vi "UHR-Fleezers Control (host) -Leonardo 04-2018 V2_sym.vi"(0 "Tab Control":T5(tab)=enum."Trap Control (RF)") -> ()   [LabVIEW 2013] (continued)
                tunnel: [w2118 w2123] -> w2110
                tunnel: w2109 -> [w2121 _]
                tunnel: w2108 -> [w2120 _]
                tunnel: w2107 -> [w2119 _]
                tunnel: w2106 -> [w2118 _]
                frame False {
                }
                frame True {
                  n1368 = Unbundle(w2131) -> (w2130:T34)
                  n1369 = call "isclickinwindow.vi"("Image Param"=w2130, "Point32"=w2129) -> ("Y px"=w2123:i32, "Height"=w2124:i32, "X px"=w2125:i32, "Width"=w2126:i32, "In image?"=w2128:bool)  [unwired: 1 in]
                  n1370 = Not(x=w2128) -> (.not. x?=w2127:bool)
                }
              }
            }
            n1371 = Not(x=w2081) -> (.not. x?=w2080:bool)
            n1372 = case shown="True" w2080 {
              tunnel: w2078 -> [_ w2144]
              tunnel: w2076 -> [_ w2143]
              tunnel: w2079 -> [_ w2142]
              tunnel: w2077 -> [_ w2141]
              frame False {
              }
              frame True {
                w2137 = FALSE ("Get Point")
                n1373 = local read "Scan lines (y)"() -> (w2146:u64)
                n1374 = local read "Actual MCL Inc (V)"() -> (w2138:dbl)
                n1375 = local read "Scan steps (MCL)"() -> (w2145:u64)
                n1376 = Divide "Y Pix/step"(x=w2141, y=w2146) -> (x/y=w2153:dbl)
                n1377 = Divide "Y V/pix"(x=w2138, y=w2153) -> (x/y=w2152:dbl)
                n1378 = Divide "Y half step offset"(x=w2138, y=2.0) -> (x/y=w2154:dbl)
                n1379 = Divide "X pix/step"(x=w2142, y=w2145) -> (x/y=w2151:dbl)
                n1380 = Negate(x=w2154) -> (-x=w2155:dbl)
                n1381 = local read "Initial Y"() -> (w2161:dbl)
                n1382 = Multiply(x=w2143, y=w2152) -> (x*y=w2162:dbl)
                n1383 = Divide "X half step offset"(x=w2138, y=2.0) -> (x/y=w2148:dbl)
                n1384 = Divide "X V/pix"(x=w2138, y=w2151) -> (x/y=w2150:dbl)
                n1385 = Multiply(x=w2138, y=w2145) -> (x*y=w2157:dbl)
                n1386 = Compound Arithmetic op=ADD(w2155, w2162, w2161) -> (w2139:dbl)
                "Pointer Y (V)" <- w2139
                n1387 = Multiply(x=w2150, y=w2144) -> (x*y=w2159:dbl)
                n1388 = Negate(x=w2148) -> (-x=w2147:dbl)
                n1389 = local read "Initial X"() -> (w2160:dbl)
                n1390 = Negate(x=w2159) -> (-x=w2158:dbl)
                n1391 = Compound Arithmetic op=ADD(w2147, w2157, w2160, w2158) -> (w2140:dbl)
                "Pointer X (V)" <- w2140
                n1392 = Or(x="Set X Only", y="Set Confocal Spot (X-Y)") -> (x .or. y?=w2133:bool)
                n1393 = Or(x="Set Confocal Spot (X-Y)", y="Set Y Only") -> (x .or. y?=w2132:bool)
                n1394 = case shown="True" w2133 {
                  tunnel: w2140 -> [_ w2163]
                  frame False {
                  }
                  frame True {
                    n1395 = property on="AO2" class="Slide (strict)"("Val(Sgnl)"=w2163) -> ()  [unwired: 2 in, 2 out]
                  }
                }
                n1396 = case shown="True" w2132 {
                  tunnel: w2139 -> [_ w2164]
                  frame False {
                  }
                  frame True {
                    n1397 = property on="AO1" class="Slide (strict)"("Val(Sgnl)"=w2164) -> ()  [unwired: 2 in, 2 out]
                  }
                }
                n1398 = local write "Set Confocal Spot (X-Y)"(w2137) -> ()
                n1399 = local write "Set X Only"(w2137) -> ()
                n1400 = local write "Set Y Only"(w2137) -> ()
              }
            }
          }
          frame 3 {
            n1401 = local read "BD 2 Frequency 1 (MHz)"() -> (w2165:dbl)
            n1402 = local read "BD 1 Frequency 1 (MHz)"() -> (w2166:dbl)
            n1403 = local write "Manipulating Trap"(TRUE ("Manipulating Trap")) -> ()
            n1404 = local write "Coords"(T8 {"Horizontal"=0, "Vertical"=0} ("Coords")) -> ()
            n1405 = while {
              tunnel: w2171 -> [w2176]
              tunnel: w2169 -> [w2175]
              tunnel: w2167 -> [w2174]
              tunnel: w2166 -> [w2173]
              tunnel: w2165 -> [w2172]
              stop <- w2177 stop-if-true
              n1406 = event shown="[0] \"Pane\": Mouse Move" {
                selector: _ -> [_ _]
                dyn-events: _ -> [_ _]
                timeout: _ -> [_ _]
                tunnel: ["Force Manip Abort" w2241] -> w2177
                tunnel: w2176 -> [w2184 _]
                tunnel: w2175 -> [w2182 _]
                tunnel: w2174 -> [w2181 _]
                tunnel: w2173 -> [w2180 _]
                tunnel: w2172 -> [w2179 _]
                event Mouse Move {
                  n1407 = event-data() -> ("Time"=w2185:u32, "Coords"=w2186:T8)  [unwired: 3 out]
                  n1408 = Less?(x=w2185, y=w2184) -> (x < y?=w2183:bool)
                  n1409 = case "Makes sure old motion events prior to mouse click aren't used" shown="False" w2183 {
                    tunnel: w2186 -> [w2228 _]
                    tunnel: w2182 -> [w2229 _]
                    tunnel: w2181 -> [w2206 _]
                    tunnel: w2180 -> [w2202 _]
                    tunnel: w2179 -> [w2201 _]
                    frame False {
                      n1410 = Subtract(x=w2228, y=w2229) -> (x-y=w2227:T8)
                      "Coords" <- w2227
                      n1411 = local read "Y RF Frequency Limits (MHz)"() -> (w2187:T16)
                      n1412 = To Double Precision Float(number=w2227) -> (double precision float=w2226:cluster{"Horizontal":dbl, "Vertical":dbl})
                      n1413 = Multiply(x=cluster{"Horizontal":dbl, "Vertical":dbl} {"Horizontal"=-1.0, "Vertical"=1.0}, y="Manipulation Scaling") -> (x*y=w2222:cluster{"Horizontal":dbl, "Vertical":dbl})
                      n1414 = local read "X RF Frequency Limits (MHz)"() -> (w2188:T16)
                      n1415 = Multiply(x=w2226, y=w2222) -> (x*y=w2224:cluster{"Horizontal":dbl, "Vertical":dbl})
                      n1416 = Unbundle By Name(w2224) -> ("Horizontal"=w2219:dbl, "Vertical"=w2223:dbl)
                      n1417 = Unbundle By Name(w2187) -> ("Maximum"=w2190:dbl, "Minimum"=w2189:dbl)
                      n1418 = Boolean To (0,1)(Boolean="Manip. X?") -> (0, 1=w2217:i16)
                      n1419 = Boolean To (0,1)(Boolean="Manip. Y?") -> (0, 1=w2214:i16)
                      n1420 = local read "BD 1 Frequency 2 (MHz)"() -> (w2204:dbl)
                      n1421 = Multiply(x=w2223, y=w2214) -> (x*y=w2216:dbl)
                      n1422 = Multiply(x=w2217, y=w2219) -> (x*y=w2220:dbl)
                      n1423 = local read "BD 2 Frequency 2 (MHz)"() -> (w2203:dbl)
                      n1424 = Unbundle By Name(w2188) -> ("Maximum"=w2192:dbl, "Minimum"=w2191:dbl)
                      n1425 = Add(x=w2201, y=w2216) -> (x+y=w2194:dbl)
                      n1426 = Add(x=w2202, y=w2220) -> (x+y=w2196:dbl)
                      n1427 = In Range and Coerce(upper limit=w2192, x=w2196, lower limit=w2191) -> (coerced(x)=w2195:dbl)  [unwired: 1 out]
                      n1428 = In Range and Coerce(upper limit=w2190, x=w2194, lower limit=w2189) -> (coerced(x)=w2193:dbl)  [unwired: 1 out]
                      n1429 = Subtract(x=w2195, y=w2204) -> (x-y=w2213:dbl)
                      n1430 = Subtract(x=w2193, y=w2203) -> (x-y=w2212:dbl)
                      n1431 = Square(x=w2213) -> (x^2=w2211:dbl)
                      n1432 = Square(x=w2212) -> (x^2=w2210:dbl)
                      n1433 = Add(x=w2211, y=w2210) -> (x+y=w2209:dbl)
                      n1434 = Square Root(x=w2209) -> (sqrt(x)=w2205:dbl)
                      n1435 = In Range and Coerce(upper limit="Limit Max (MHz)", x=w2205, lower limit="Limit Min (MHz)") -> (In Range?=w2198:bool)  [unwired: 1 out]
                      n1436 = Not(x="Limits Enable") -> (.not. x?=w2197:bool)
                      n1437 = Or(x=w2198, y=w2197) -> (x .or. y?=w2199:bool)
                      n1438 = case shown="True" w2199 {
                        tunnel: w2206 -> [_ w2239]
                        tunnel: w2205 -> [_ w2230]
                        tunnel: w2195 -> [_ w2237]
                        tunnel: w2204 -> [_ w2236]
                        tunnel: w2193 -> [_ w2235]
                        tunnel: w2203 -> [_ w2234]
                        tunnel: w2188 -> [_ w2232]
                        tunnel: w2187 -> [_ w2231]
                        frame False {
                        }
                        frame True {
                          n1439 = local read "BD 1 Frequency 3 (MHz)"() -> (w2238:dbl)
                          n1440 = local read "BD 2 Frequency 3 (MHz)"() -> (w2233:dbl)
                          n1441 = local write "Trap Delta (MHz)"(w2230) -> ()
                          n1442 = property on="Initial delta (MHz)" class="DigNum (strict)"("Val(Sgnl)"=w2230) -> ()  [unwired: 2 in, 2 out]
                          n1443 = call "set RF board frequency - interlace.vi"("Board 2 Frequency Limits"=w2231, "Board 1 Frequency Limits"=w2232, "FPGA VI Reference In"=w2239, "Board 2 Frequency 3 (MHz)"=w2233, "Board 1 Frequency 3 (MHz)"=w2238, "Board 2 Frequency 2 (MHz)"=w2234, "Board 2 Frequency 1 (MHz)"=w2235, "Board 1 Frequency 2 (MHz)"=w2236, "Board 1 Frequency 1  (MHz)"=w2237) -> ()  [unwired: 1 in, 2 out]
                          n1444 = local write "BD 2 Frequency 1 (MHz)"(w2235) -> ()
                          n1445 = local write "BD 1 Frequency 1 (MHz)"(w2237) -> ()
                        }
                      }
                    }
                    frame True {
                    }
                  }
                }
                event Mouse Up {
                  n1446 = event-data() -> ("Button"=w2240:u16)  [unwired: 8 out]
                  n1447 = case shown="3" w2240 {
                    tunnel: [FALSE TRUE] -> w2241
                    frame 0, Default {
                    }
                    frame 3 {
                      n1448 = local write "Manipulating Trap"(FALSE ("Manipulating Trap")) -> ()
                    }
                  }
                }
              }
            }
          }
        }
      }
      event Mouse Move {
        n1449 = event-data() -> ()  [unwired: 6 out]
      }
    }
    n1450 = local read "Stop All"() -> (w2062:bool)
    n1451 = node-c288() -> ()  [unwired: 2 out]
  }
  n1452 = node-c288(w53) -> ()  [unwired: 1 out]
  n1453 = node-c288(w102) -> ()  [unwired: 1 out]
  n1454 = node-c288(w109) -> ()  [unwired: 1 out]
  n1455 = node-c288(i64 1 ("Period"), 1 ("Processor")) -> (w195:T25)  [unwired: 2 out]
  n1456 = timed-loop "Acquire Data" {
    tunnel: w61 -> [w2550]
    tunnel: w76 -> [w2549]
    tunnel: [w2580] -> w69
    tunnel: [w2574] -> w2
    timing: w195 -> [_]
    timing-out: [_] -> w194
    tunnel: w93 -> [w2396]
    stop <- "Stop All" stop-if-true
    (unwired) u32 0 ("Number of Elements")
    w2383 = "NI_ChannelName" ("name")
    n1457 = node-c288() -> ()  [unwired: 2 out]
    n1458 = First Call?() -> (First Call?: T/F=w2349:bool)
    n1459 = Or(x="Reset", y=w2349) -> (x .or. y?=w2350:bool)
    n1460 = local read "MCL Tracking"() -> (w2287:bool)
    n1461 = case "Reset data stream" shown="True" w2350 {
      tunnel: w2550 -> [w2700 w2708]
      tunnel: w2549 -> [w2699 w2707]
      tunnel: [w2700 w2702] -> w2285
      tunnel: [w2699 w2701] -> w2545
      frame False {
      }
      frame True {
        w2705 = TRUE ("AI to FIFO")
        n1462 = local write "Overflow (data lost)"(FALSE ("Overflow (data lost)")) -> ()
        n1463 = call "reset FPGA DMA.vi"("error in"=w2707, "FPGA VI Reference In"=w2708) -> ("error out"=w2703:errorcluster, "FPGA VI Reference Out"=w2704:T20)
        n1464 = xnode "Read/Write Control"("FPGA VI Reference In"=w2704, "error in"=w2703, "AI to FIFO"=w2705, "APD to FIFO"=w2705) -> ("FPGA VI Reference Out"=w2702:T20, "error out"=w2701:errorcluster)
      }
    }
    n1465 = Or(x="Start AOD Scan", y="Trap Raster Scan") -> (x .or. y?=w2503:bool)
    n1466 = case "Start AOM raster scan" shown="True" w2503 {
      tunnel: w2285 -> [w3441 w3452]
      tunnel: w2545 -> [w3440 w3451]
      tunnel: [w3441 w3445] -> w2284
      tunnel: [w3440 w3444] -> w2544
      frame False {
      }
      frame True {
        n1467 = case shown="True" "Restart DMA? (AOD)" {
          tunnel: [w3492 w3494] -> w3446
          tunnel: [w3491 w3493] -> w3447
          tunnel: w3452 -> [w3492 w3496]
          tunnel: w3451 -> [w3491 w3495]
          frame False {
          }
          frame True {
            n1468 = local write "Overflow (data lost)"(FALSE ("Overflow (data lost)")) -> ()
            n1469 = call "reset FPGA DMA.vi"("error in"=w3495, "FPGA VI Reference In"=w3496) -> ("error out"=w3493:errorcluster, "FPGA VI Reference Out"=w3494:T20)
          }
        }
        n1470 = local write "Trap Raster Scan"(FALSE ("Trap Raster Scan")) -> ()
        n1471 = case shown="False" "Move MCL Also?" {
          tunnel: w3447 -> [w3456 w3486]
          tunnel: w3446 -> [w3457 w3487]
          tunnel: [w3455 w3490] -> w3445
          tunnel: [w3454 w3489] -> w3444
          tunnel: "Raster to target force?" -> [w3453 w3459]
          frame False {
            w3458 = TRUE ("AI to FIFO")
            n1472 = xnode "Read/Write Control"("FPGA VI Reference In"=w3457, "error in"=w3456, "AI to FIFO"=w3458, "APD to FIFO"=w3458, "Start scan"=w3458, "Raster to target force"=w3453) -> ("FPGA VI Reference Out"=w3455:T20, "error out"=w3454:errorcluster)
          }
          frame True {
            w3483 = FALSE ("1D or 2D Scan?")
            w3488 = TRUE ("AI to FIFO")
            # "Count for MCL loop"
            # "N total cycles"
            # "N steps"
            # "V_int"
            n1473 = local read "Scan Range (nm)"() -> (w3465:dbl)
            n1474 = local read "Number of F/B Scans (AOD)"() -> (w3482:u16)
            n1475 = Sign(1:w3465) -> (0:w3464:dbl)
            n1476 = Compound Arithmetic op=MULTIPLY(w3465, "MCL Step Position Ratio", "MCL/AOM Scale Tweak") -> (w3469:dbl)
            n1477 = Negate(x=w3464) -> (-x=w3461:dbl)
            n1478 = Multiply(x=w3461, y="MCL Step Increment (V_int)") -> (x*y=w3463:dbl)
            n1479 = Divide(x=w3469, y="MCL X Cal (nm/V)") -> (x/y=w3475:dbl)
            n1480 = Multiply(x=32767.0 ("y"), y=w3475) -> (x*y=w3481:dbl)
            n1481 = local read "Total Counts (ticks)"() -> (w3466:u32)
            n1482 = local read "Cycles/step (AOD)"() -> (w3477:u64)
            n1483 = local read "Scan steps (AOD)"() -> (w3478:u64)
            n1484 = Divide(x=w3481, y=10.0) -> (x/y=w3474:dbl)
            n1485 = Divide(x=w3474, y="MCL Step Increment (V_int)") -> (x/y=w3472:dbl)
            n1486 = Absolute Value(x=w3472) -> (abs(x)=w3460:dbl)
            n1487 = Compound Arithmetic op=MULTIPLY(w3478, w3477, w3466) -> (w3473:u64)
            n1488 = local write "wait to reset values"(w3488) -> ()
            n1489 = local write "MCL Scanning"(w3488) -> ()
            n1490 = Divide(x=w3473, y=w3460) -> (x/y=w3470:dbl)
            "MCL Count" <- w3470
            n1491 = xnode "Read/Write Control"("FPGA VI Reference In"=w3487, "error in"=w3486, "Scan steps (MCL)"=w3460, "Number of scans (MCL)"=w3482, "Cycles per step (MCL)"=u64 1, "Scan freq.  increment (MCL)"=w3463, "1D or 2D Scan?"=w3483, "MCL Scan Axis"=w3483, "Cont. Scan (MCL)"=w3483, "MCL count"=w3470) -> ("FPGA VI Reference Out"=w3485:T20, "error out"=w3484:errorcluster)
            n1492 = xnode "Read/Write Control"("FPGA VI Reference In"=w3485, "error in"=w3484, "AI to FIFO"=w3488, "APD to FIFO"=w3488, "Start scan"=w3488, "Start scan (MCL)"=w3488, "Raster to target force"=w3459) -> ("FPGA VI Reference Out"=w3490:T20, "error out"=w3489:errorcluster)
          }
        }
        "Raster Scanning..." <- TRUE ("Scanning...")
      }
    }
    n1493 = And(x="Save scans", y=w2503) -> (x .and. y?=w2543:bool)
    n1494 = Compound Arithmetic op=OR("Start MCL Scan", "Confocal Image", "Confocal Linescan") -> (w2501:bool)
    n1495 = And(x="Save Data (MCL)", y=w2501) -> (x .and. y?=w2542:bool)
    n1496 = case "Start MCL raster scan" shown="True" w2501 {
      tunnel: w2284 -> [w2991 w3006]
      tunnel: w2544 -> [w2990 w3005]
      tunnel: [w2991 w3001] -> w2319
      tunnel: [w2990 w3000] -> w2318
      tunnel: [FALSE w2999] -> w2528
      tunnel: "Start MCL Scan" -> [_ w2994]
      tunnel: "Confocal Image" -> [_ w2993]
      tunnel: "Confocal Linescan" -> [_ _]
      frame False {
      }
      frame True {
        w2999 = TRUE
        n1497 = case shown="True" "Restart DMA? (MCL)" {
          tunnel: [w3051 w3053] -> w3004
          tunnel: [w3050 w3052] -> w3003
          tunnel: w3006 -> [w3051 w3056]
          tunnel: w3005 -> [w3050 w3055]
          frame False {
          }
          frame True {
            n1498 = call "reset FPGA DMA.vi"("error in"=w3055, "FPGA VI Reference In"=w3056) -> ("error out"=w3052:errorcluster, "FPGA VI Reference Out"=w3053:T20)
            n1499 = local write "Overflow (data lost)"(FALSE ("Overflow (data lost)")) -> ()
          }
        }
        n1500 = case shown="False" w2994 {
          selector: w2994 -> [_ w3010]
          tunnel: w2993 -> [w3009 _]
          tunnel: [w3009 w3010] -> w2992
          frame False {
            n1501 = property on="2D or 1D Scan" class="Bool (strict)"("Val(Sgnl)"=w3009) -> ()  [unwired: 2 in, 2 out]
            n1502 = property on="Confocal Image" class="Bool (strict)"("Value"=FALSE ("Start Confocal Map")) -> ()  [unwired: 2 in, 2 out]
          }
          frame True {
          }
        }
        n1503 = local write "MCL Scanning"(w2999) -> ()
        n1504 = local read "AO1"() -> (w2996:dbl)
        n1505 = local read "AO2"() -> (w2995:dbl)
        n1506 = case shown="True" "Center Scan" {
          tunnel: w3004 -> [w3017 w3049]
          tunnel: w3003 -> [w3016 w3048]
          tunnel: [w3015 w3047] -> w3001
          tunnel: [w3014 w3046] -> w3000
          tunnel: [w3012 w3033] -> w2998
          tunnel: [w3011 w3032] -> w2997
          tunnel: w2996 -> [w3012 w3038]
          tunnel: w2995 -> [w3011 w3041]
          tunnel: w2992 -> [_ _]
          frame False {
            w3013 = TRUE ("AI to FIFO")
            n1507 = xnode "Read/Write Control"("FPGA VI Reference In"=w3017, "error in"=w3016, "AI to FIFO"=w3013, "APD to FIFO"=w3013, "Start scan (MCL)"=w3013) -> ("FPGA VI Reference Out"=w3015:T20, "error out"=w3014:errorcluster)
          }
          frame True {
            w3045 = TRUE ("AI to FIFO")
            n1508 = local read "Scan steps (MCL)"() -> (w3024:u64)
            n1509 = local read "Scan lines (y)"() -> (w3020:u64)
            n1510 = local read "Fast Scan Dir"() -> (w3031:bool)
            n1511 = local read "Actual MCL Inc (V)"() -> (w3021:dbl)
            n1512 = Decrement(x=w3020) -> (x-1=w3019:u64)
            n1513 = Decrement(x=w3024) -> (x-1=w3023:u64)
            n1514 = Multiply(x=w3021, y=w3019) -> (x*y=w3018:dbl)
            n1515 = Divide(x=w3018, y=2.0) -> (x/y=w3028:dbl)
            n1516 = Multiply(x=w3021, y=w3023) -> (x*y=w3022:dbl)
            n1517 = Divide(x=w3022, y=2.0) -> (x/y=w3027:dbl)
            n1518 = Select(t=w3027, s=w3031, f=w3028) -> (s? t:f=w3026:dbl)
            n1519 = Select(t=w3028, s=w3031, f=w3027) -> (s? t:f=w3030:dbl)
            n1520 = Subtract(x=w3038, y=w3030) -> (x-y=w3029:dbl)
            n1521 = Subtract(x=w3041, y=w3026) -> (x-y=w3025:dbl)
            n1522 = local read "2D or 1D Scan"() -> (w3043:bool)
            n1523 = Not(x=w3031) -> (.not. x?=w3037:bool)
            n1524 = Not(x=w3043) -> (.not. x?=w3039:bool)
            n1525 = And(x=w3031, y=w3039) -> (x .and. y?=w3040:bool)
            n1526 = And(x=w3039, y=w3037) -> (x .and. y?=w3042:bool)
            n1527 = Select(t=w3041, s=w3042, f=w3025) -> (s? t:f=w3032:dbl)
            n1528 = Select(t=w3038, s=w3040, f=w3029) -> (s? t:f=w3033:dbl)
            n1529 = call "Volt to I16.vi"("Voltage In"=w3033) -> ("I16 Voltage Out"=w3036:i16)
            n1530 = call "Volt to I16.vi"("Voltage In"=w3032) -> ("I16 Voltage Out"=w3035:i16)
            n1531 = xnode "Read/Write Control"("FPGA VI Reference In"=w3049, "error in"=w3048, "AI to FIFO"=w3045, "APD to FIFO"=w3045, "Start scan (MCL)"=w3045, "AO1 (Y)"=w3036, "AO2 (X)"=w3035) -> ("FPGA VI Reference Out"=w3047:T20, "error out"=w3046:errorcluster)
          }
        }
        "Initial Y" <- w2998
        "Initial X" <- w2997
        "wait to reset values" <- w2999
      }
    }
    n1532 = local read "Trap Pos Elements/DMA read"() -> (w2392:u32)
    n1533 = local read "Trap AI Elements/DMA read"() -> (w2317:u32)
    n1534 = local read "APD Elements/DMA read"() -> (w2431:u32)
    n1535 = local read "Trap AI FIFO Depth"() -> (w2590:u32)
    n1536 = xnode "Invoke Method"("FPGA VI Reference In"=w2319, "error in"=w2318, "Number of Elements"=w2392, "Timeout (ms)"=-1) -> ("Data"=w2356:u16[], "Elements Remaining"=→"Trap Pos FIFO El Remaining":u32)  [unwired: 2 out]
    n1537 = xnode "Invoke Method"("FPGA VI Reference In"=w2319, "error in"=w2318, "Number of Elements"=w2317, "Timeout (ms)"=-1 ("Timeout")) -> ("FPGA VI Reference Out"=w2288:T20, "error out"=w2320:errorcluster, "Data"=w2316:i16[], "Elements Remaining"=w2321:u32)
    "Trap AI FIFO El. Rem." <- w2321
    n1538 = xnode "Get APD Data"("FPGA VI Reference In"=w2319, "error in"=w2318, "Number of Elements"=w2431, "Timeout (ms)"=-1) -> ("Data"=w2430:u32[], "Elements Remaining"=→"APD FIFO Elements Remaining":u32)  [unwired: 2 out]
    n1539 = Subtract(x=w2590, y=w2317) -> (x-y=w2589:u32)
    n1540 = Decimate 1D Array(w2356) -> (w2353:u16[], w2355:u16[], w2354:u16[])
    n1541 = Divide(x=w2321, y=w2589) -> (x/y=w2588:dbl)
    "Buffer Status" <- w2588
    n1542 = To Unsigned Long Integer(number=w2353) -> (unsigned 32bit integer=w2352:u32[])
    n1543 = Join Numbers(hi=w2355, lo=w2354) -> ((hi.lo)=w2351:u32[])
    n1544 = Equal?(x=w2588, y=1.0) -> (x = y?=w2586:bool)
    n1545 = Join Numbers(hi=w2352, lo=w2351) -> ((hi.lo)=w2345:u64[])
    n1546 = call "IR AOM word to freq - vec.vi"("Frequency Word In (double vec)"=w2345) -> ("Frequency Out"=w2391:dbl[])
    n1547 = case "Alert buffer overflow" shown="True" w2586 {
      frame False {
      }
      frame True {
        n1548 = call <vilib>:"Beep.vi"() -> ()  [unwired: 3 in, 9 out]
        "Overflow (data lost)" <- TRUE ("Overflow (data lost)")
      }
    }
    n1549 = Decimate 1D Array(w2391) -> (w2390:dbl[], w2389:dbl[])
    n1550 = Array Size(array=w2316) -> (size(s)=→"Waveform Chart":i32)
    n1551 = Build Array(w2390, w2389) -> (w2388:dbl[][])
    n1552 = local read "Trap Sets"() -> (w2463:u32)
    n1553 = case "Deinterlace trap data, average down PSD" shown="2" w2463 {
      tunnel: w2316 -> [w3086 w3151]
      tunnel: [w3083 w3148] -> w2456
      tunnel: [w3086 w3150] -> w2348
      tunnel: "Detector Type" -> [w3085 w3146]
      tunnel: [w3084 w3149] -> w2455
      tunnel: [w3082 w3147] -> w2561
      frame 1, Default {
        n1554 = Divide(x=w3086, y=3276.7) -> (x/y=w3087:dbl[])
        n1555 = Decimate 1D Array(w3087) -> (w3096:dbl[], w3095:dbl[], w3094:dbl[], w3093:dbl[], w3092:dbl[], w3091:dbl[], w3090:dbl[], w3089:dbl[])
        n1556 = case shown="\"IR-QPD + PSD + FB-QPD position\"" w3085 {
          tunnel: w3096 -> [w3120 w3145]
          tunnel: w3095 -> [w3119 w3144]
          tunnel: w3094 -> [w3104 w3122]
          tunnel: w3093 -> [w3105 w3132]
          tunnel: w3092 -> [w3118 w3143]
          tunnel: w3091 -> [w3117 w3142]
          tunnel: w3090 -> [w3101 w3123]
          tunnel: w3089 -> [w3100 w3121]
          tunnel: [w3099 w3129] -> w3084
          tunnel: [w3098 w3128] -> w3083
          tunnel: [w3097 w3127] -> w3082
          frame "IR-QPD + PSD + FB-QPD", Default {
            w3097 = 0  # Channel pattern
            n1557 = Divide(x=w3120, y=w3105) -> (x/y=w3107:dbl[])
            n1558 = Divide(x=w3119, y=w3105) -> (x/y=w3106:dbl[])
            n1559 = Divide(x=w3118, y=w3101) -> (x/y=w3103:dbl[])
            n1560 = Divide(x=w3117, y=w3100) -> (x/y=w3102:dbl[])
            n1561 = Build Array(w3107, w3106, w3105, w3104, w3103, w3102, w3101, w3100) -> (w3098:dbl[][])
            n1562 = Bundle("T1 Y", "T1 X", "T1 Sum", "FB Sum", "PSD Y", "PSD X", "PSD Y Sum", "PSD X Sum") -> (w3116:T42)  [unwired: 1 out]
            n1563 = Cluster To Array(cluster=w3116) -> (array=w3099:string[])
          }
          frame "IR-QPD + PSD + FB-QPD position" {
            w3127 = 3  # Channel pattern
            n1564 = Negate(x=w3123) -> (-x=w3124:dbl[])
            n1565 = Divide(x=w3145, y=w3132) -> (x/y=w3134:dbl[])
            n1566 = Divide(x=w3144, y=w3132) -> (x/y=w3133:dbl[])
            n1567 = Divide(x=w3143, y=w3123) -> (x/y=w3131:dbl[])
            n1568 = Divide(x=w3142, y=w3124) -> (x/y=w3130:dbl[])
            n1569 = Build Array(w3134, w3133, w3132, w3121, w3122, w3131, w3130, w3123) -> (w3128:dbl[][])
            n1570 = Bundle("T1 Y", "T1 X", "T1 Sum", "FB X", "FB Sum", "PSD Y", "PSD X", "PSD Y Sum") -> (w3141:T42)  [unwired: 1 out]
            n1571 = Cluster To Array(cluster=w3141) -> (array=w3129:string[])
          }
        }
      }
      frame 2 {
        n1572 = case shown="\"UCB Fleezers 052511\"" w3146 {
          tunnel: w3151 -> [w3213 w3280 w3319 w3419]
          tunnel: [w3152 w3272 w3315 w3350] -> w3150
          tunnel: [w3179 w3263 w3317 w3397] -> w3149
          tunnel: [w3178 w3227 w3308 w3364] -> w3148
          tunnel: [w3172 w3262 w3349 w3395] -> w3147
          frame "IR-QPD + PSD + FB-QPD", Default {
            w3172 = 1  # Channel pattern
            # "time average x2 the 4th signal and the 4 psd signals (detection laser)"
            # "deinterlace 3 signals from qpd"
            n1573 = Decimate 1D Array(w3213) -> (w3212:i16[], w3211:i16[], w3177:i16[], w3210:i16[], w3200:i16[], w3198:i16[], w3197:i16[], w3195:i16[])
            n1574 = call "downsample 1D array - double.vi"("Ave N"=2.0, "Array In"=w3200) -> ("Array Out"=w3199:dbl[])  [unwired: 1 out]
            n1575 = call "downsample 1D array - double.vi"("Ave N"=2.0, "Array In"=w3195) -> ("Array Out"=w3194:dbl[])  [unwired: 1 out]
            n1576 = call "downsample 1D array - double.vi"("Ave N"=2.0, "Array In"=w3197) -> ("Array Out"=w3196:dbl[])  [unwired: 1 out]
            n1577 = call "downsample 1D array - double.vi"("Ave N"=2.0, "Array In"=w3198) -> ("Array Out"=w3180:dbl[])  [unwired: 1 out]
            n1578 = Decimate 1D Array(w3212) -> (w3209:i16[], w3181:i16[])
            n1579 = Decimate 1D Array(w3211) -> (w3208:i16[], w3206:i16[])
            n1580 = Decimate 1D Array(w3210) -> (w3207:i16[], w3205:i16[])
            n1581 = Decimate 1D Array(w3177) -> (w3176:i16[], w3175:i16[])
            n1582 = Interleave 1D Arrays(w3209, w3208, w3207, w3181, w3206, w3205, w3176, w3175, w3199, w3180, w3196, w3194) -> (w3193:dbl[])
            n1583 = To Word Integer(number=w3193) -> (16bit integer=w3152:i16[])
            n1584 = Divide(x=w3193, y=3276.7) -> (x/y=w3192:dbl[])
            n1585 = Decimate 1D Array(w3192) -> (w3191:dbl[], w3190:dbl[], w3189:dbl[], w3188:dbl[], w3187:dbl[], w3186:dbl[], w3174:dbl[], w3173:dbl[], w3185:dbl[], w3184:dbl[], w3183:dbl[], w3182:dbl[])
            n1586 = Divide(x=w3191, y=w3189) -> (x/y=w3159:dbl[])
            n1587 = Divide(x=w3190, y=w3189) -> (x/y=w3158:dbl[])
            n1588 = Divide(x=w3188, y=w3186) -> (x/y=w3157:dbl[])
            n1589 = Divide(x=w3187, y=w3186) -> (x/y=w3156:dbl[])
            n1590 = Divide(x=w3185, y=w3183) -> (x/y=w3155:dbl[])
            n1591 = Divide(x=w3184, y=w3182) -> (x/y=w3154:dbl[])
            n1592 = Bundle("T1 Y", "T1 X", "T1 Sum", "T2 Y", "T2 X", "T2 Sum", "T1 FB Sum", "T2 FB Sum", "PSD Y", "PSD X", "PSD Y Sum", "PSD X Sum") -> (w3160:T43)  [unwired: 1 out]
            n1593 = Build Array(w3159, w3158, w3189, w3157, w3156, w3186, w3174, w3173, w3155, w3154, w3183, w3182) -> (w3178:dbl[][])
            n1594 = Cluster To Array(cluster=w3160) -> (array=w3179:string[])
          }
          frame "IR-QPD + PSD + FB-QPD X position" {
            w3262 = 2  # Channel pattern
            # "convert\nADC numbers\nto volts"
            # "time average x2 the 3 psd signals (detection laser)"
            # "deinterlace 3 signals from qpds"
            n1595 = Decimate 1D Array(w3280) -> (w3279:i16[], w3278:i16[], w3215:i16[], w3216:i16[], w3225:i16[], w3222:i16[], w3219:i16[], w3250:i16[])
            n1596 = Decimate 1D Array(w3279) -> (w3277:i16[], w3264:i16[])
            n1597 = call "downsample 1D array - I16.vi"("Ave N"=2.0, "Array In"=w3225) -> ("Array Out"=w3223:i16[])  [unwired: 1 in]
            n1598 = call "downsample 1D array - I16.vi"("Ave N"=2.0, "Array In"=w3222) -> ("Array Out"=w3220:i16[])  [unwired: 1 in]
            n1599 = Decimate 1D Array(w3278) -> (w3276:i16[], w3274:i16[])
            n1600 = Decimate 1D Array(w3216) -> (w3275:i16[], w3273:i16[])
            n1601 = Decimate 1D Array(w3250) -> (w3249:i16[], w3247:i16[])
            n1602 = Decimate 1D Array(w3215) -> (w3248:i16[], w3246:i16[])
            n1603 = call "downsample 1D array - I16.vi"("Ave N"=2.0, "Array In"=w3219) -> ("Array Out"=w3217:i16[])  [unwired: 1 in]
            n1604 = Interleave 1D Arrays(w3277, w3276, w3275, w3264, w3274, w3273, w3249, w3248, w3247, w3246, w3223, w3220, w3217) -> (w3272:i16[])
            n1605 = Divide(x=w3272, y=3276.7) -> (x/y=w3271:dbl[])
            n1606 = Decimate 1D Array(w3271) -> (w3270:dbl[], w3269:dbl[], w3268:dbl[], w3267:dbl[], w3266:dbl[], w3265:dbl[], w3238:dbl[], w3236:dbl[], w3235:dbl[], w3233:dbl[], w3232:dbl[], w3231:dbl[], w3228:dbl[])
            n1607 = Divide(x=w3270, y=w3268) -> (x/y=w3254:dbl[])
            n1608 = Divide(x=w3269, y=w3268) -> (x/y=w3253:dbl[])
            n1609 = Divide(x=w3267, y=w3265) -> (x/y=w3252:dbl[])
            n1610 = Divide(x=w3266, y=w3265) -> (x/y=w3251:dbl[])
            n1611 = Divide(x=w3238, y=w3236) -> (x/y=w3237:dbl[])
            n1612 = Divide(x=w3235, y=w3233) -> (x/y=w3234:dbl[])
            n1613 = Divide(x=w3232, y=w3228) -> (x/y=w3230:dbl[])
            n1614 = Negate(x=w3228) -> (-x=w3226:dbl[])
            n1615 = Divide(x=w3231, y=w3226) -> (x/y=w3229:dbl[])
            n1616 = Bundle("T1 Y", "T1 X", "T1 Sum", "T2 Y", "T2 X", "T2 Sum", "T1 FB X", "T1 FB Sum", "T2 FB X", "T2 FB Sum", "PSD Y", "PSD X", "PSD Y Sum") -> (w3255:T44)  [unwired: 1 out]
            n1617 = Build Array(w3254, w3253, w3268, w3252, w3251, w3265, w3237, w3236, w3234, w3233, w3230, w3229, w3228) -> (w3227:dbl[][])
            n1618 = Cluster To Array(cluster=w3255) -> (array=w3263:string[])
          }
          frame "UCB Fleezers 052511" {
            w3349 = 2  # Channel pattern
            n1619 = Select(t=i16 -1, s="Negate X signals", f=i16 1) -> (s? t:f=w3289:i16)
            n1620 = Decimate 1D Array(w3319) -> (w3290:i16[], w3291:i16[], w3302:i16[], w3318:i16[], w3287:i16[], w3285:i16[], w3283:i16[], w3299:i16[])
            n1621 = Multiply(x=w3289, y=w3291) -> (x*y=w3288:i16[])
            n1622 = Decimate 1D Array(w3290) -> (w3347:i16[], w3337:i16[])
            n1623 = Decimate 1D Array(w3288) -> (w3346:i16[], w3345:i16[])
            n1624 = Decimate 1D Array(w3302) -> (w3296:i16[], w3295:i16[])
            n1625 = Decimate 1D Array(w3318) -> (w3301:i16[], w3300:i16[])
            n1626 = Decimate 1D Array(w3285) -> (w3284:i16[])  [unwired: 1 out]
            n1627 = Decimate 1D Array(w3299) -> (w3298:i16[], w3297:i16[])
            n1628 = Decimate 1D Array(w3283) -> (w3282:i16[])  [unwired: 1 out]
            n1629 = Decimate 1D Array(w3287) -> (w3286:i16[])  [unwired: 1 out]
            n1630 = Interleave 1D Arrays(w3347, w3346, w3301, w3337, w3345, w3300, w3298, w3296, w3297, w3295, w3286, w3284, w3282) -> (w3315:i16[])
            n1631 = Divide(x=w3315, y=3276.7) -> (x/y=w3344:dbl[])
            n1632 = Decimate 1D Array(w3344) -> (w3343:dbl[], w3342:dbl[], w3341:dbl[], w3340:dbl[], w3339:dbl[], w3338:dbl[], w3314:dbl[], w3312:dbl[], w3311:dbl[], w3309:dbl[], w3307:dbl[], w3304:dbl[], w3305:dbl[])
            n1633 = Divide(x=w3343, y=w3341) -> (x/y=w3324:dbl[])
            n1634 = Divide(x=w3342, y=w3341) -> (x/y=w3323:dbl[])
            n1635 = Divide(x=w3340, y=w3338) -> (x/y=w3322:dbl[])
            n1636 = Divide(x=w3339, y=w3338) -> (x/y=w3321:dbl[])
            n1637 = Divide(x=w3314, y=w3312) -> (x/y=w3313:dbl[])
            n1638 = Divide(x=w3311, y=w3309) -> (x/y=w3310:dbl[])
            n1639 = Divide(x=w3307, y=w3305) -> (x/y=w3306:dbl[])
            n1640 = Divide(x=w3304, y=w3305) -> (x/y=w3303:dbl[])
            n1641 = Build Array(w3324, w3323, w3341, w3322, w3321, w3338, w3313, w3312, w3310, w3309, w3306, w3303, w3305) -> (w3308:dbl[][])
            n1642 = Bundle("T1 Y", "T1 X", "T1 Sum", "T2 Y", "T2 X", "T2 Sum", "T1 FB X", "T2 FB Sum", "T2 FB X", "T2 FB Sum", "PSD Y", "PSD X", "PSD Sum") -> (w3325:T44)  [unwired: 1 out]
            n1643 = Cluster To Array(cluster=w3325) -> (array=w3317:string[])
          }
          frame "IR-QPD + PSD + FB-QPD XY positions" {
            w3395 = 4  # Channel pattern
            # "time average x2 the 3 psd signals (detection laser)"
            # "deinterlace 3 signals from qpds"
            n1644 = Decimate 1D Array(w3419) -> (w3418:i16[], w3417:i16[], w3396:i16[], w3416:i16[], w3362:i16[], w3408:i16[], w3407:i16[], w3384:i16[])
            n1645 = Decimate 1D Array "QPD Y"(w3418) -> (w3415:i16[], w3398:i16[])
            n1646 = call "downsample 1D array - double.vi"("Ave N"=2.0, "Array In"=w3408) -> ("Array Out"=w3383:dbl[])  [unwired: 1 out]
            n1647 = call "downsample 1D array - double.vi"("Ave N"=2.0, "Array In"=w3407) -> ("Array Out"=w3382:dbl[])  [unwired: 1 out]
            n1648 = Decimate 1D Array "Feedback Sum"(w3396) -> (w3380:i16[], w3378:i16[])
            n1649 = Decimate 1D Array "Feedback Y"(w3362) -> (w3361:i16[], w3360:i16[])
            n1650 = Decimate 1D Array "Feedback X"(w3384) -> (w3381:i16[], w3379:i16[])
            n1651 = Decimate 1D Array "QPD Sum"(w3416) -> (w3413:i16[], w3411:i16[])
            n1652 = Decimate 1D Array "QPD X"(w3417) -> (w3414:i16[], w3412:i16[])
            n1653 = Interleave 1D Arrays(w3415, w3414, w3413, w3398, w3412, w3411, w3361, w3381, w3380, w3360, w3379, w3378, w3383, w3382) -> (w3406:dbl[])
            n1654 = To Word Integer(number=w3406) -> (16bit integer=w3350:i16[])
            n1655 = Divide(x=w3406, y=3276.7) -> (x/y=w3405:dbl[])
            n1656 = Decimate 1D Array(w3405) -> (w3404:dbl[], w3403:dbl[], w3402:dbl[], w3401:dbl[], w3400:dbl[], w3399:dbl[], w3357:dbl[], w3371:dbl[], w3355:dbl[], w3356:dbl[], w3369:dbl[], w3353:dbl[], w3367:dbl[], w3365:dbl[])
            n1657 = Divide(x=w3404, y=w3402) -> (x/y=w3388:dbl[])
            n1658 = Divide(x=w3403, y=w3402) -> (x/y=w3387:dbl[])
            n1659 = Divide(x=w3401, y=w3399) -> (x/y=w3386:dbl[])
            n1660 = Divide(x=w3400, y=w3399) -> (x/y=w3385:dbl[])
            n1661 = Divide(x=w3357, y=w3355) -> (x/y=w3354:dbl[])
            n1662 = Divide(x=w3371, y=w3355) -> (x/y=w3370:dbl[])
            n1663 = Divide(x=w3356, y=w3353) -> (x/y=w3352:dbl[])
            n1664 = Divide(x=w3369, y=w3353) -> (x/y=w3368:dbl[])
            n1665 = Negate(x=w3365) -> (-x=w3363:dbl[])
            n1666 = Divide(x=w3367, y=w3363) -> (x/y=w3366:dbl[])
            n1667 = Bundle("T1 Y", "T1 X", "T1 Sum", "T2 Y", "T2 X", "T2 Sum", "T1 FB Y", "T1 FB X", "T1 FB Sum", "T2 FB Y", "T2 FB X", "T2 FB Sum", "PSD X", "PSD Y Sum") -> (w3351:T45)  [unwired: 1 out]
            n1668 = Build Array(w3388, w3387, w3402, w3386, w3385, w3399, w3354, w3370, w3355, w3352, w3368, w3353, w3366, w3365) -> (w3364:dbl[][])
            n1669 = Cluster To Array(cluster=w3351) -> (array=w3397:string[])
          }
        }
      }
    }
    "AI labels" <- w2455
    n1670 = xnode "Read/Write Control"("FPGA VI Reference In"=w2288) -> ("FPGA VI Reference Out"=w2281:T20, "BD1 Frequency Out 1"=w2302:u64)  [unwired: 1 in, 1 out]
    n1671 = local read "BD 1 Frequency 2 (MHz)"() -> (w2293:dbl)
    n1672 = To Double Precision Float(number=w2302) -> (double precision float=w2299:dbl)
    n1673 = Multiply(x=49125000.0, y=6.0) -> (x*y=w2298:dbl)
    n1674 = Multiply(x=w2299, y=w2298) -> (x*y=w2296:dbl)
    n1675 = Scale By Power Of 2(n=-48, x=w2296) -> (x*2^n=w2295:dbl)
    n1676 = local read "Dynamic Force FB"() -> (w2292:bool)
    n1677 = local read "Trap Pos. FB ON"() -> (w2291:bool)
    n1678 = Divide(x=w2295, y=1000000.0) -> (x/y=w2286:dbl)
    n1679 = case shown="True" w2287 {
      tunnel: w2286 -> [_ w2677]
      tunnel: w2284 -> [_ w2664]
      frame False {
      }
      frame True {
        n1680 = local read "AOM X Cal (nm/MHz)"() -> (w2674:dbl)
        n1681 = local read "Zero T1 position"() -> (w2676:dbl)
        n1682 = Subtract(x=w2677, y=w2676) -> (x-y=w2675:dbl)
        n1683 = Multiply(x=w2675, y=w2674) -> (x*y=w2673:dbl)
        n1684 = local read "MCL X Cal (nm/V)"() -> (w2670:dbl)
        n1685 = Multiply(x=w2673, y="Tracking factor") -> (x*y=w2671:dbl)
        n1686 = local read "Zero MCL x position"() -> (w2669:dbl)
        n1687 = Divide(x=w2671, y=w2670) -> (x/y=w2668:dbl)
        n1688 = Add(x=w2669, y=w2668) -> (x+y=w2661:dbl)
        "Current MCL (V)" <- w2661
        n1689 = Multiply(x=w2661, y=32767.0) -> (x*y=w2665:dbl)
        n1690 = Divide(x=w2665, y=10.0) -> (x/y=w2662:dbl)
        n1691 = To Word Integer(number=w2662) -> (16bit integer=w2663:i16)
        n1692 = xnode "Read/Write Control"("FPGA VI Reference In"=w2664, "AO2 (X)"=w2663) -> ()  [unwired: 1 in, 2 out]
      }
    }
    n1693 = Subtract(x=w2293, y=w2286) -> (x-y=w2282:dbl)
    "Current deltaFreq" <- w2282
    n1694 = Compound Arithmetic op=AND(w2292, w2291, "Real time offset \ncorrection for setpoint") -> (w2289:bool)
    n1695 = case shown="True" w2289 {
      tunnel: w2282 -> [_ w2680]
      tunnel: w2281 -> [_ w2679]
      frame False {
      }
      frame True {
        n1696 = local read "T1 kappa_x (pN/nm)"() -> (w2688:dbl)
        n1697 = local read "T1 alpha_x (nm/V)"() -> (w2689:dbl)
        n1698 = local read "Negate offset difference"() -> (w2690:bool)
        n1699 = local read "Offset file step size"() -> (w2698:dbl)
        n1700 = Multiply(x="Target Force (pN)", y=2.0) -> (x*y=w2686:dbl)
        n1701 = local read "Setpoint offset\nCorrection values"() -> (w2695:dbl[])
        n1702 = Divide(x=w2680, y=w2698) -> (x/y=w2697:dbl)
        n1703 = Select(t=-1, s=w2690, f=1) -> (s? t:f=w2691:i32)
        n1704 = To Long Integer(number=w2697) -> (32bit integer=w2696:i32)
        n1705 = Multiply(x=w2689, y=w2688) -> (x*y=w2685:dbl)
        n1706 = Divide(x=w2686, y=w2685) -> (x/y=w2684:dbl)
        n1707 = Index Array(array=w2695, index=w2696) -> (element=w2694:dbl)
        n1708 = Multiply(x=w2691, y=w2694) -> (x*y=w2683:dbl)
        n1709 = Add(x=w2684, y=w2683) -> (x+y=w2682:dbl)
        n1710 = To Fixed-Point(number=w2682) -> (fixed-point=w2678:fxp<+/-,16,1>)  [unwired: 1 in]
        "Actual setpoint" <- w2678
        n1711 = xnode "Read/Write Control"("FPGA VI Reference In"=w2679, "Trap Pos. FB SP"=w2678) -> ()  [unwired: 1 in, 2 out]
      }
    }
    n1712 = case shown="True" "Take full offset\n data for display" {
      tunnel: [w2647 w2653] -> w2480
      tunnel: [w2646 w2652] -> w2478
      tunnel: w2282 -> [_ w2659]
      frame False {
        n1713 = Divide(x="T2 offset_x (mV)", y=1000.0) -> (x/y=w2646:dbl)
        n1714 = Divide(x="T1 offset_x (mV)", y=1000.0) -> (x/y=w2647:dbl)
      }
      frame True {
        n1715 = local read "Offset Values"() -> (w2660:T14)
        n1716 = local read "Offset file step size"() -> (w2658:dbl)
        n1717 = Unbundle By Name(w2660) -> ("Trap 1X offset"=w2655:dbl[], "Trap 2X offset"=w2654:dbl[])
        n1718 = Divide(x=w2659, y=w2658) -> (x/y=w2657:dbl)
        n1719 = To Long Integer(number=w2657) -> (32bit integer=w2656:i32)
        n1720 = Index Array(array=w2655, index=w2656) -> (element=w2653:dbl)
        n1721 = Index Array(array=w2654, index=w2656) -> (element=w2652:dbl)
      }
    }
    n1722 = Decimate 1D Array(w2430) -> (w2453:u32[], w2398:u32[])
    n1723 = local read "DMA Update Period (s)"() -> (w2464:dbl)
    n1724 = local read "BD 1 Frequency 2 (MHz)"() -> (w2340:dbl)
    n1725 = local read "BD 1 Frequency 1 (MHz)"() -> (w2341:dbl)
    n1726 = Build Array(w2453, w2398) -> (w2525:u32[][])
    n1727 = local read "Data Period (s)"() -> (w2443:dbl)
    n1728 = Decimate 1D Array(w2348) -> (w2371:i16[], w2370:i16[], w2368:i16[], w2367:i16[])  [unwired: 9 out]
    n1729 = To Double Precision Float(number=w2525) -> (double precision float=w2526:dbl[][])
    n1730 = local read "APD Integration Time (s)"() -> (w2411:dbl)
    n1731 = Divide(x=w2371, y=w2370) -> (x/y=w2372:dbl[])
    n1732 = Divide(x=w2368, y=w2367) -> (x/y=w2369:dbl[])
    n1733 = feedback #1(0.0) -> (w2385:dbl)
    n1734 = Add(x=w2464, y=w2385) -> (x+y=w2563:dbl)
    n1735 = feedback-in #1(w2563) -> ()
    n1736 = local read "AOM X Cal (nm/MHz)"() -> (w2338:dbl)
    n1737 = To Time Stamp(1:w2385) -> (0:w2384:timestamp)
    n1738 = Split 1D Array(array=w2372, index="N El. to Ave.") -> (second subarray=w2375:dbl[])  [unwired: 1 out]
    n1739 = Split 1D Array(array=w2369, index="N El. to Ave.") -> (second subarray=w2374:dbl[])  [unwired: 1 out]
    n1740 = local read "Trap X AI1 (DMA)"() -> (w2373:T13)
    n1741 = Multiply(x=w2443, y="Trap Disp. Downsample") -> (x*y=w2386:dbl)
    "Display Period (s)" <- w2386
    n1742 = Bundle("BD 1 Frequency 1 (MHz)"=w2341, "BD 1 Frequency 2 (MHz)"=w2340) -> (w2342:T46)  [unwired: 1 out]
    n1743 = for "Trap AI" {
      tunnel: [w3081] -> w2557 mode=indexing
      tunnel: w2384 -> [w3071]
      tunnel: "Trap Disp. Downsample" -> [w3079]
      tunnel: w2456 -> [w3077] mode=indexing
      tunnel: w2443 -> [w3076]
      tunnel: w2455 -> [w3075] mode=indexing
      tunnel: w2383 -> [w3074]
      tunnel: [w3073] -> w2422 mode=indexing
      tunnel: w2386 -> [w3072]
      n1744 = Bundle By Name("Y"=w3077, "dt"=w3076) -> (w3078:waveform(dbl))  [unwired: 1 out]
      n1745 = Set Waveform Attribute(5:w3075, 6:w3074, 7:w3078) -> (3:w3073:waveform(dbl))  [unwired: 1 in, 2 out]
      n1746 = call "downsample 1D array - double.vi"("Ave N"=w3079, "Array In"=w3077) -> ("Array Out"=w3080:dbl[])  [unwired: 1 out]
      n1747 = Bundle By Name(cluster=w3073, "t0"=w3071, "Y"=w3080, "dt"=w3072) -> (w3081:waveform(dbl))
    }
    n1748 = call-poly <vilib>:"Mean.vi"("X"=w2374) -> ("mean"=w2362:dbl)  [unwired: 1 out]
    n1749 = call-poly <vilib>:"Mean.vi"("X"=w2375) -> ("mean"=w2363:dbl)  [unwired: 1 out]
    n1750 = Cluster To Array(cluster=w2342) -> (array=w2339:dbl[])
    n1751 = Reciprocal(x=w2386) -> (1/x=→"Trap Disp. Freq. (Hz)":dbl)
    n1752 = local read "Data points/scans (MCL)"() -> (w2537:dbl)
    n1753 = To Fixed-Point(number=w2362) -> (fixed-point=w2360:fxp<+/-,16,1>)  [unwired: 1 in]
    n1754 = To Fixed-Point(number=w2363) -> (fixed-point=w2361:fxp<+/-,16,1>)  [unwired: 1 in]
    n1755 = Bundle("Trap 1 Pos.", "Trap 2 Pos.") -> (w2382:cluster{string, string})  [unwired: 1 out]
    n1756 = Bundle By Name(cluster=w2373, "Set 1"=w2361, "Set 2"=w2360) -> (→"Trap X AI1 (DMA)":T13)
    n1757 = Cluster To Array(cluster=w2382) -> (array=w2379:string[])
    n1758 = for "Trap Position" {
      tunnel: w2388 -> [w2721] mode=indexing
      tunnel: "Trap Disp. Downsample" -> [w2720]
      tunnel: w2386 -> [w2718]
      tunnel: w2384 -> [w2717]
      tunnel: w2383 -> [w2715]
      tunnel: w2379 -> [w2714] mode=indexing
      tunnel: [w2713] -> w2337 mode=indexing
      tunnel: w2339 -> [w2711] mode=indexing
      tunnel: w2338 -> [w2709]
      n1759 = call "downsample 1D array - double.vi"("Ave N"=w2720, "Array In"=w2721) -> ("Array Out"=w2719:dbl[])  [unwired: 1 out]
      n1760 = Subtract(x=w2719, y=w2711) -> (x-y=w2712:dbl[])
      n1761 = Multiply(x=w2709, y=w2712) -> (x*y=w2710:dbl[])
      n1762 = Bundle By Name("Y"=w2710, "dt"=w2718, "t0"=w2717) -> (w2716:waveform(dbl))  [unwired: 1 out]
      n1763 = Set Waveform Attribute(5:w2714, 6:w2715, 7:w2716) -> (3:w2713:waveform(dbl))  [unwired: 1 in, 2 out]
    }
    "Trap Positions" <- w2337
    n1764 = Bundle("APD 1", "APD 2") -> (w2556:cluster{string, string})  [unwired: 1 out]
    n1765 = Cluster To Array(cluster=w2556) -> (array=w2553:string[])
    n1766 = for "APD" {
      tunnel: w2526 -> [w3060] mode=indexing
      tunnel: w2411 -> [w3068]
      tunnel: [w3064] -> w2418 mode=indexing
      tunnel: "APD Disp. Scale" -> [w3065]
      tunnel: w2383 -> [w3063]
      tunnel: w2553 -> [w3062] mode=indexing
      tunnel: "APD Disp. Downsample" -> [w3058]
      tunnel: [w3061] -> w2552
      tunnel: w2384 -> [w3057]
      n1767 = call "integrate 1D array interval - double.vi"("Ave N"=w3058, "Array In"=w3060) -> ("Array Out"=w3059:dbl[])  [unwired: 1 out]
      n1768 = Multiply(x=w3068, y=w3058) -> (x*y=w3061:dbl)
      n1769 = Divide(x=w3059, y=w3065) -> (x/y=w3066:dbl[])
      n1770 = Bundle By Name("t0"=w3057, "Y"=w3066, "dt"=w3061) -> (w3067:waveform(dbl))  [unwired: 1 out]
      n1771 = Set Waveform Attribute(5:w3062, 6:w3063, 7:w3067) -> (3:w3064:waveform(dbl))  [unwired: 1 in, 2 out]
    }
    "APD Display Period (s)" <- w2552
    n1772 = Reciprocal(x=w2552) -> (1/x=→"APD Display Freq. (Hz)":dbl)
    n1773 = local read "Display Period (s)"() -> (w2442:dbl)
    n1774 = Increment(x=w2537) -> (x+1=w2538:dbl)
    n1775 = Index Array(array=w2337, index=0) -> (element=w2335:waveform(dbl))
    n1776 = To Double Precision Float(number=w2453) -> (double precision float=w2452:dbl[])
    n1777 = feedback #2(w2538) -> (w2541:dbl)
    n1778 = Select(t=0, s=w2528, f=w2541) -> (s? t:f=w2534:dbl)
    n1779 = Array Size(array=w2452) -> (size(s)=w2540:i32)
    n1780 = Add(x=w2540, y=w2534) -> (x+y=w2535:dbl)
    n1781 = Unbundle By Name(w2335) -> ("Y"=w2333:dbl[])
    n1782 = feedback #3(w2453) -> (w2524:u32[])
    n1783 = Build Array (concatenate)(w2524, w2453) -> (w2521:u32[])
    n1784 = feedback #4(w2398) -> (w2417:u32[])
    n1785 = Divide(x="Bead Sep. Int. Time (s)", y=w2442) -> (x/y=w2331:dbl)
    n1786 = Build Array (concatenate)(w2417, w2398) -> (w2416:u32[])
    n1787 = Greater?(x=w2535, y=w2537) -> (0:w2536:bool)
    n1788 = feedback #5(w2333) -> (w2334:dbl[])
    n1789 = Build Array (concatenate)(w2333, w2334) -> (w2332:dbl[])
    n1790 = Select(t=w2534, s=w2536, f=w2535) -> (s? t:f=w2533:dbl)
    n1791 = feedback-in #2(w2533) -> ()
    n1792 = Array Size(array=w2521) -> (size(s)=w2518:i32)
    n1793 = Array Size(array=w2453) -> (size(s)=w2520:i32)
    n1794 = local read "MCL Scanning"() -> (w2531:bool)
    n1795 = local read "APD Integration Time (s)"() -> (w2425:dbl)
    n1796 = Build Array (concatenate)(w2418, w2557) -> (w2420:waveform(dbl)[])
    "All Signals" <- w2420
    n1797 = Split 1D Array(array=w2332, index=w2331) -> (first subarray=w2325:dbl[])  [unwired: 1 out]
    n1798 = feedback-in #5(w2325) -> ()
    n1799 = Multiply(x=w2520, y="APD Ave N") -> (x*y=w2519:dbl)
    n1800 = Greater?(x=w2518, y=w2519) -> (0:w2522:bool)
    n1801 = Not(x=w2536) -> (.not. x?=w2530:bool)
    n1802 = To Double Precision Float(number=w2398) -> (double precision float=w2397:dbl[])
    n1803 = call-poly <vilib>:"Mean.vi"("X"=w2325) -> ("mean"=w2324:dbl)  [unwired: 1 out]
    "Mean T1 Position (nm)" <- w2324
    n1804 = Subtract(x=w2325, y=w2324) -> (x-y=w2330:dbl[])
    n1805 = Square(x=w2330) -> (x^2=w2329:dbl[])
    n1806 = And(x=w2530, y=w2531) -> (x .and. y?=w2532:bool)
    n1807 = call-poly <vilib>:"Mean.vi"("X"=w2329) -> ("mean"=w2328:dbl)  [unwired: 1 out]
    n1808 = case shown="True" w2522 {
      tunnel: w2521 -> [w2841 w2848]
      tunnel: [w2841 w2846] -> w2469
      tunnel: w2519 -> [_ w2843]
      tunnel: w2518 -> [_ w2847]
      tunnel: w2416 -> [w2840 w2845]
      tunnel: [w2840 w2842] -> w2413
      frame False {
      }
      frame True {
        n1809 = Subtract(x=w2847, y=w2843) -> (x-y=w2844:dbl)
        n1810 = Array Subset(array=w2848, index=w2844, length=w2843) -> (w2846:u32[])
        n1811 = Array Subset(array=w2845, index=w2844, length=w2843) -> (w2842:u32[])
      }
    }
    n1812 = feedback-in #3(w2469) -> ()
    n1813 = feedback-in #4(w2413) -> ()
    n1814 = Or(x=w2532, y=w2528) -> (x .or. y?=w2529:bool)
    n1815 = Square Root(x=w2328) -> (sqrt(x)=w2327:dbl)
    n1816 = Equal?(x="Tab Control 6", y=T36."High Res Display") -> (x = y?=w2459:bool)
    n1817 = Multiply(x="APD Disp. Scale", y=w2418) -> (x*y=w2427:waveform(dbl)[])
    n1818 = Multiply(x="APD Disp. Downsample", y=w2425) -> (x*y=w2423:dbl)
    n1819 = Multiply(x=10.0, y=w2327) -> (x*y=→"Trap 1 Position RMS (A)":dbl)
    n1820 = Divide(x=w2427, y=w2423) -> (x/y=w2395:waveform(dbl)[])
    n1821 = Index Array(array=w2395, index=0) -> (element=w2405:waveform(dbl))
    n1822 = case "For computing FFTs for display" shown="True" "Compute FFT" {
      tunnel: w2422 -> [_ w3525]
      frame False {
      }
      frame True {
        n1823 = Build Array("FFT 1 Choice 1", "FFT 1 Choice 2", "FFT 2 Choice 1", "FFT 2 Choice 2") -> (w3518:u16[])
        n1824 = Array Size(array=w3525) -> (size(s)=w3524:i32)
        n1825 = feedback-in #6(w3518) -> ()
        n1826 = feedback #6(u16[] [100, 100, 100, 100]) -> (w3519:u16[])
        n1827 = feedback-in #7("# Spectra to Ave.") -> ()
        n1828 = feedback #7("# Spectra to Ave.") -> (w3516:dbl)
        n1829 = Not Equal?(x="# Spectra to Ave.", y=w3516) -> (x != y?=w3515:bool)
        n1830 = Not Equal?(x=w3518, y=w3519) -> (x != y?=w3517:bool)
        n1831 = feedback #8(1.0) -> (w3502:dbl)
        n1832 = Compound Arithmetic op=OR("Reset FFT", w3517, w3515) -> (w3500:bool)
        n1833 = Select(t=1.0, s=w3500, f=w3502) -> (s? t:f=w3504:dbl)
        n1834 = Greater?(x=w3504, y="# Spectra to Ave.") -> (0:w3523:bool)
        n1835 = Increment(x=w3504) -> (x+1=w3503:dbl)
        n1836 = feedback-in #8(w3503) -> ()
        n1837 = local read "DMA Update Period (s)"() -> (w3498:dbl)
        n1838 = Multiply(x="# Spectra to Ave.", y=w3498) -> (x*y=→"Ave. Time (s)":dbl)
        n1839 = Build Array(cluster{"f0":dbl, "df":dbl, "magnitude":dbl[]} {"f0"=0.0, "df"=0.0, "magnitude"=[]} ("PSD")) -> (w3507:cluster{"f0":dbl, "df":dbl, "magnitude":dbl[]}[])
        n1840 = Build Array(w3507, w3507, w3507, w3507) -> (w3509:T47)
        n1841 = feedback #9(w3509) -> (w3514:T47)
        n1842 = for {
          N: 4 -> [_]
          tunnel: w3518 -> [w3547] mode=indexing
          tunnel: w3525 -> [w3548]
          tunnel: w3524 -> [w3550]
          tunnel: w3500 -> [w3543]
          tunnel: w3523 -> [w3542]
          tunnel: "# Spectra to Ave." -> [w3541]
          tunnel: [w3540] -> w3513 mode=indexing
          tunnel: w3514 -> [w3545] mode=indexing
          tunnel: [w3544] -> w3501 mode=indexing
          tunnel: w3504 -> [w3539]
          n1843 = Less?(x=w3547, y=w3550) -> (x < y?=w3549:bool)
          n1844 = Index Array(array=w3548, index=w3547) -> (element=w3546:waveform(dbl))
          n1845 = case shown="True" w3549 {
            tunnel: w3546 -> [_ w3567]
            tunnel: w3545 -> [w3552 w3565]
            tunnel: [w3552 w3553] -> w3544
            tunnel: w3543 -> [_ w3564]
            tunnel: w3542 -> [_ w3557]
            tunnel: w3541 -> [_ w3556]
            tunnel: [cluster{"f0":dbl, "df":dbl, "magnitude":dbl[]} {"f0"=0.0, "df"=0.0, "magnitude"=[]} ("PSD") w3558] -> w3540
            tunnel: w3539 -> [_ w3555]
            frame False {
            }
            frame True {
              n1846 = call <vilib>:"Std Deviation and Variance.vi"("X"=w3567) -> ("mean"=w3568:dbl)  [unwired: 1 in, 2 out]
              n1847 = Subtract(x=w3567, y=w3568) -> (x-y=w3566:waveform(dbl))
              n1848 = xnode "Spectral Measurements"("Signals"=w3566) -> ("PSD"=w3560:cluster{"f0":dbl, "df":dbl, "magnitude":dbl[]})  [unwired: 1 in, 1 out]
              n1849 = case shown="False" w3564 {
                tunnel: w3565 -> [w3577 _]
                tunnel: [w3573 w3582] -> w3553
                tunnel: w3560 -> [w3576 w3583]
                tunnel: w3557 -> [w3575 _]
                frame False {
                  n1850 = Build Array (concatenate)(w3577, w3576) -> (w3574:cluster{"f0":dbl, "df":dbl, "magnitude":dbl[]}[])
                  n1851 = case shown="True" w3575 {
                    tunnel: w3574 -> [w3578 w3581]
                    tunnel: [w3578 w3579] -> w3573
                    frame False {
                    }
                    frame True {
